vi "Close Panel.vi"(8 "error in (no error)":errorcluster, 10 "ArrayPanel":refnum<class "ArrayPanel.lvclass">, 11 "2DArrayManager in":refnum<class "2DArrayManager.lvclass">) -> (0 "error out":errorcluster, 3 "2DArrayManager out":refnum<class "2DArrayManager.lvclass">)   [LabVIEW 2020, in "OOPanel.lvlib" / "2DArrayManager.lvclass"]
uses:
  2DArrayManager.lvclass
  ArrayPanel/ArrayPanel.lvclass
  C:/dev/lv20CE/lv-oopanel/OOPanel/Panel/Panel.lvclass
  2DArrayManager.lvclass/2DArrayManager.ctl
  Manager/Manager.lvclass
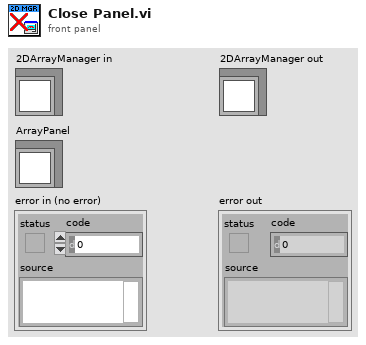
[diagram p1: front panel]
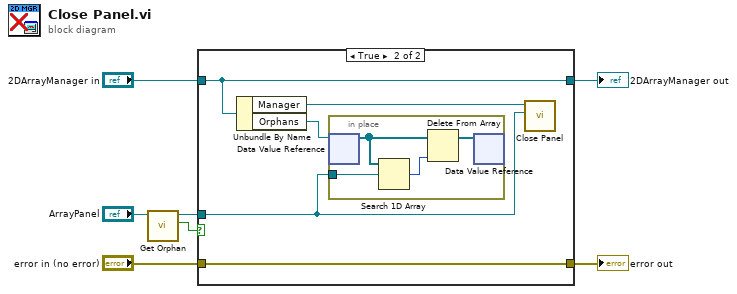
[diagram p0: block diagram]
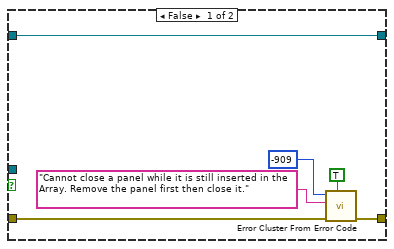
[diagram p2: hidden frame]
diagram:
  n1 = call "Get Orphan.vi"("ArrayPanel in"="ArrayPanel") -> ("Orphan"=w6:bool, "ArrayPanel out"=w5:refnum<class "ArrayPanel.lvclass">)  [unwired: 8 in, 1 out]
  n2 = case shown="True" w6 {
    tunnel: w5 -> [_ w15]
    tunnel: "2DArrayManager in" -> [w9 w18]
    tunnel: "error in (no error)" -> [w13 w14]
    tunnel: [w9 w18] -> w2
    tunnel: [w8 w14] -> w1
    frame False {
      n3 = call <vilib>:"Error Cluster From Error Code.vi"("show call chain? (False)"=TRUE, "error in (no error)"=w13, "error message (\"\")"="Cannot close a panel while it is still inserted in the Array. Remove the panel first then close it." ("error message (\"\")"), "error code (0)"=-909) -> ("error out"=w8:errorcluster)  [unwired: 5 in]
    }
    frame True {
      n4 = Unbundle By Name(w18) -> ("Manager"=w16:refnum<class "Manager.lvclass">, "Orphans"=w17:refnum<data-value>)
      n5 = in-place {
        in-place-border: w15 -> [w22]
        n6 = in-place-dvr #1(w17) -> (w21:refnum<class "ArrayPanel.lvclass">[])  [unwired: 1 out]
        n7 = Search 1D Array(1D array=w21, element=w22) -> (index of element=w20:i32)  [unwired: 1 in]
        n8 = Delete From Array(array=w21, index=w20) -> (array with subset deleted=w19:refnum<class "ArrayPanel.lvclass">[])  [unwired: 1 in, 1 out]
        n9 = in-place-dvr #1(w19) -> ()  [unwired: 2 out]
      }
      n10 = call "Close Panel.vi"("Panel"=w15, "Manager in"=w16) -> ()  [unwired: 8 in, 2 out]
    }
  }
  "error out" <- w1
  "2DArrayManager out" <- w2
